vi "Cron Next (Jenkins-compatible).vi"(7 "Job Name":string="* * * ? *", 9 "Nb Occurences (min: 1)":u16=1 min=1, 10 "Reference timestamp (Now)":timestamp, 11 "Cron Expression":string="* * * ? *") -> (1 "Occurences":timestamp[](array[timestamp]), 2 "Next Occurence":timestamp, 3 "syntax valid?":bool)   [LabVIEW 2013, in "openCron.lvlib"]
uses:
  openCron.lvlib
  Cron.Jenkins/Cron.Jenkins.lvclass
  Cron.Jenkins/Cron.Jenkins.lvclass/Cron.Jenkins.ctl
  Cron/Cron.lvclass
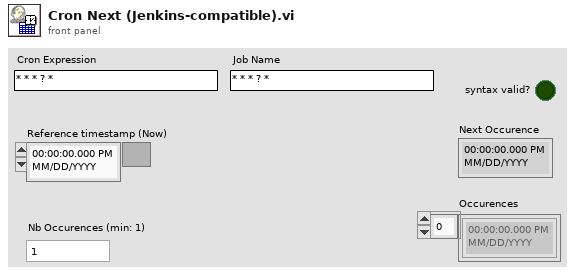
[diagram p1: front panel]
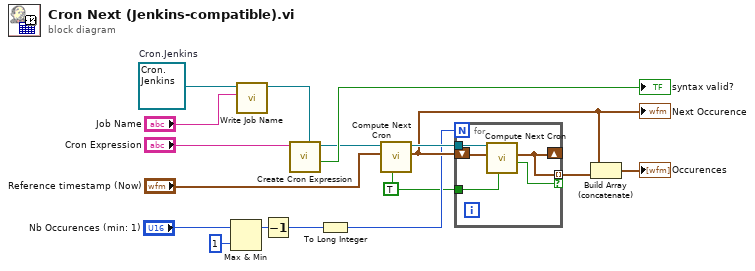
[diagram p0: block diagram]
diagram:
  w3 = refnum<class "Cron.Jenkins.lvclass"> refnum  # Cron.Jenkins
  w4 = TRUE ("Ignore DST?")
  n1 = Max & Min(x="Nb Occurences (min: 1)", y=u16 1) -> (max(x,y)=w10:u16)  [unwired: 1 out]
  n2 = call "Write Job Name.vi"("Job Name"="Job Name", "Cron.Jenkins in"=w3) -> ("Cron.Jenkins out"=w2:refnum<class "Cron.Jenkins.lvclass">)  [unwired: 8 in, 1 out]
  n3 = Decrement(x=w10) -> (x-1=w9:u16)
  n4 = call "Create Cron Expression.vi"("Cron in"=w2, "Cron Expression"="Cron Expression") -> ("expression valid"=→"syntax valid?":bool, "Cron out"=w15:refnum<class "Cron.Jenkins.lvclass">)  [unwired: 7 in, 1 out]
  n5 = To Long Integer(number=w9) -> (32bit integer=w5:i32)
  n6 = call "Compute Next Cron.vi"("Ignore DST?"=w4, "Time Stamp (Now)"="Reference timestamp (Now)", "Cron in"=w15) -> ("Next Occurence"=w7:timestamp, "Cron out"=w13:refnum<class "Cron.Jenkins.lvclass">)  [unwired: 5 in, 2 out]
  "Next Occurence" <- w7
  n7 = for {
    N: w5 -> [_]
    shift-right: [w20] -> _
    shift-left: w7 -> [w22]
    tunnel: w13 -> [w21]
    tunnel: [w20] -> w8 mode=indexing if=w18
    tunnel: w4 -> [w19]
    n8 = call "Compute Next Cron.vi"("Ignore DST?"=w19, "Time Stamp (Now)"=w22, "Cron in"=w21) -> ("Occurence found"=w18:bool, "Next Occurence"=w20:timestamp)  [unwired: 5 in, 2 out]
  }
  n9 = Build Array (concatenate)(w7, w8) -> (→"Occurences":timestamp[])
